vi "Initialise Interface.vi"(8 "error in (no error)":errorcluster, 10 "Initial Pump Controls":T2 {"Mass Flow SP [kg/h]" min=0.0 max=64.255}, 11 "CAN Frame Sessions":T1={"Session_Control"="Sess_Control", "Session_Params"="Sess_Params", "Session_Actuals"="Sess_Actuals", "Session_Acknowledge"="Sess_Ack", "Session_H2_Sensor"="H2_Sensor_Session", "Session_DILICO_MeasurementRequest"="Session_DILICO_MeasurementRequest", "Session_DILICO_Voltages"="Session_DILICO_Voltages"}) -> (0 "error out":errorcluster={"status"=TRUE, "code"=-1074384864, "source"="XNET Write (Signal Single-point).vi:3310001<APPEND>\n\n<b>Complete call chain:</b>\r\n     XNET Write (Signal Single-point).vi:3310001\r\n     phlair-busch-can-bus.lvlib:Initialise Interface.vi"}, 3 "output cluster":T1={"Session_Control"="Session_Control", "Session_Params"="Session_Params", "Session_Actuals"="Session_Actuals", "Session_Acknowledge"="Session_Acknowledge", "Session_H2_Sensor"="H2_Sensor_Session", "Session_DILICO_MeasurementRequest"="Session_DILICO_MeasurementRequest", "Session_DILICO_Voltages"="Session_DILICO_Voltages"})   [LabVIEW 2025, in "phlair-busch-can-bus.lvlib"]
uses:
  phlair-busch-can-bus.lvlib
  PumpControls.ctl
  CAN Frame Sessions.ctl
  <vilib>/xnet/xnet.llb/XNET Write (Signal Single-point).vi
  <userlib>/_OpenG.lib/error/error.llb/openg_error.lvlib
  <resource>/objmgr/xnet.rc
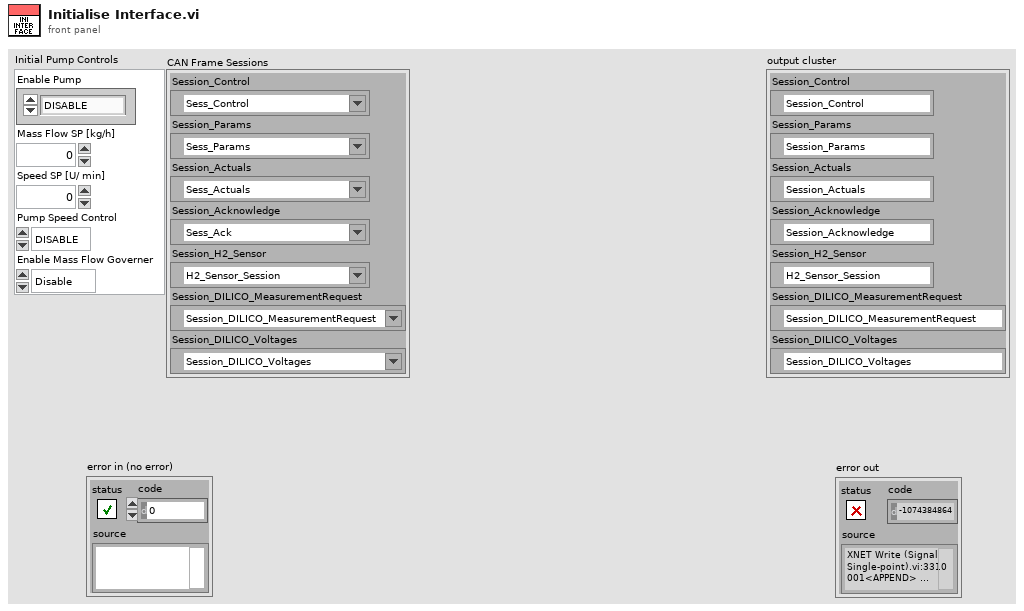
[diagram p1: front panel]
types:
  T1 = typedef "phlair-busch-can-bus.lvlib/CAN Frame Sessions.ctl" = cluster{"Session_Control":refnum<k21>, "Session_Params":refnum<k21>, "Session_Actuals":refnum<k21>, "Session_Acknowledge":refnum<k21>, "Session_H2_Sensor":refnum<k21>, "Session_DILICO_MeasurementRequest":refnum<k21>, "Session_DILICO_Voltages":refnum<k21>}
  T2 = typedef "phlair-busch-can-bus.lvlib/PumpControls.ctl" = cluster{"Enable Pump":enum16{"DISABLE", "ENABLE"}, "Mass Flow SP [kg/h]":dbl, "Speed SP [U/ min]":u16, "Pump Speed Control":enum16{"DISABLE", "ENABLE"}, "Enable Mass Flow Governer":enum8{"Disable", "Enable", "", "NA"}}
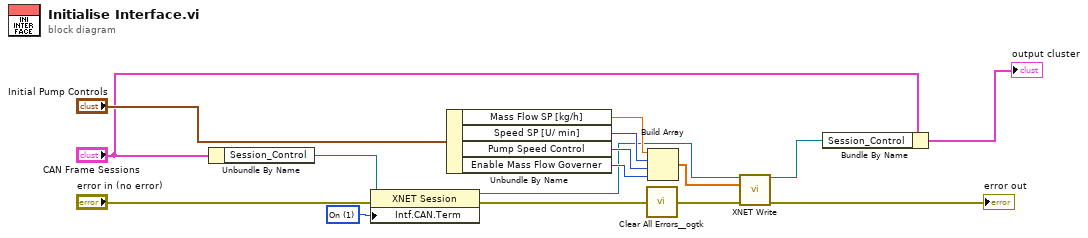
[diagram p0: block diagram]
diagram:
  w6 = u32 1 items=["Off", "On"] ("Interface:CAN:Termination")
  n1 = Unbundle By Name("CAN Frame Sessions") -> ("Session_Control"=w2:refnum<k21>)
  n2 = property class="XNET Session"(reference=w2, error in="error in (no error)", "Intf.CAN.Term"=w6) -> (reference out=w5:refnum<k21>, error out=w3:errorcluster)
  n3 = Unbundle By Name("Initial Pump Controls") -> ("Mass Flow SP [kg/h]"=w14:dbl, "Speed SP [U/ min]"=w13:u16, "Pump Speed Control"=w12:enum16{"DISABLE", "ENABLE"}, "Enable Mass Flow Governer"=w11:enum8{"Disable", "Enable", "", "NA"})
  n4 = call <userlib>:"Clear All Errors__ogtk.vi"("Error In"=w3) -> ("Error Out"=w7:errorcluster)  [unwired: 3 in]
  n5 = Build Array(w14, w13, w12, w11) -> (w1:dbl[])
  n6 = call-poly <vilib>:"XNET Write.vi"("session in"=w5, "data"=w1, "error in (no error)"=w7) -> ("session out"=w9:refnum<k21>, "error out"=→"error out":errorcluster)  [unwired: 11 in]
  n7 = Bundle By Name(cluster="CAN Frame Sessions", "Session_Control"=w9) -> (→"output cluster":T1)
